vi "Read.vi"(8 "error in (no error)":errorcluster, 11 "Boolean in":refnum<class "FPGA-Bus_FXP24_5.lvclass">) -> (0 "error out":errorcluster, 2 "Numeric":T1, 3 "Boolean out":refnum<class "FPGA-Bus_FXP24_5.lvclass">)   [LabVIEW 2021, in "FPGA-Bus_FXP24_5.lvclass"]
uses:
  FPGA-Bus_FXP24_5.lvclass
  Support/Value Type.ctl
  FPGA-Bus_FXP24_5.lvclass/FPGA-Bus_FXP24_5.ctl
  <vilib>/Utility/error.llb/Error Cluster From Error Code.vi
  <vilib>/rvi/errors/niLvFpgaAdjustHostInterfaceError.vi
  <vilib>/rvi/interface/nirviReadWriteControl/nirviReadWriteControl.xnode
  Support/FPGA Type.ctl
  NiFpgaLv.dll
  <vilib>/rvi/interface/Simulation/niFpgaSimulationCallBeginRW.vi
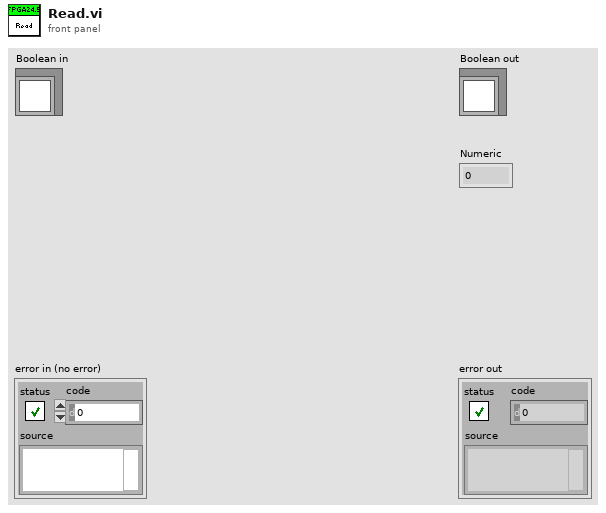
[diagram p1: front panel]
types:
  T1 = typedef "FPGA-Bus_FXP24_5.lvclass/Value Type.ctl" = dbl
  T2 = typedef "FPGA-Bus_FXP24_5.lvclass/FPGA Type.ctl" = refnum<k20>
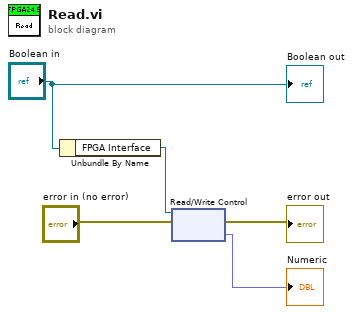
[diagram p0: block diagram]
diagram:
  n1 = Unbundle By Name("Boolean in") -> ("FPGA Interface"=w3:T2)
  n2 = xnode "Read/Write Control"("FPGA VI Reference In"=w3, "error in"="error in (no error)") -> ("error out"=→"error out":errorcluster, "Value"=→"Numeric":fxp<+/-,24,5>)  [unwired: 1 out]
  "Boolean out" <- "Boolean in"
